vi "Operaciones Boleanas.vi"() -> ()   [LabVIEW 2022 SP3]
panel:
  out "AND COMPOUND":bool
  out "AND EN CASCADA":bool
  in  "Boton A 9":bool
  in  "Boton A 8":bool
  in  "Boton A 7":bool
  in  "Boton A 6":bool
  in  "Boton A 5":bool
  in  "Boton A 4":bool
  in  "Boton A 3":bool
  in  "Boton A 2":bool
  out "NAND":bool
  out "NOR":bool
  out "OR":bool
  out "AND":bool
  in  "Boton B":bool
  in  "Boton A":bool
  # "GATE AND Y OR"
  # "ESTA SOLUCION NOS DA UN RESULTADO PARA LO \n8 RESULTADOS , ES DECIR SI TODOS SON CERO LA \nCOMPUERTA AND TE DA CERO Y SI TODOS ESTAN \nEN 1 LA COMPUERTA AND TE DA 1"
  # "COMPOUND ARITMETIC"
  # "CON ESTA FUNCION PARA AHORRAR MEMORIA SE PUEDE USAR EL COMPUND \nARIMETMETIC QUE TE RESUMEN LAS OPERACIONES BOLEANAS QUE QUIERES\nEN UN SOLO BLOQUE"
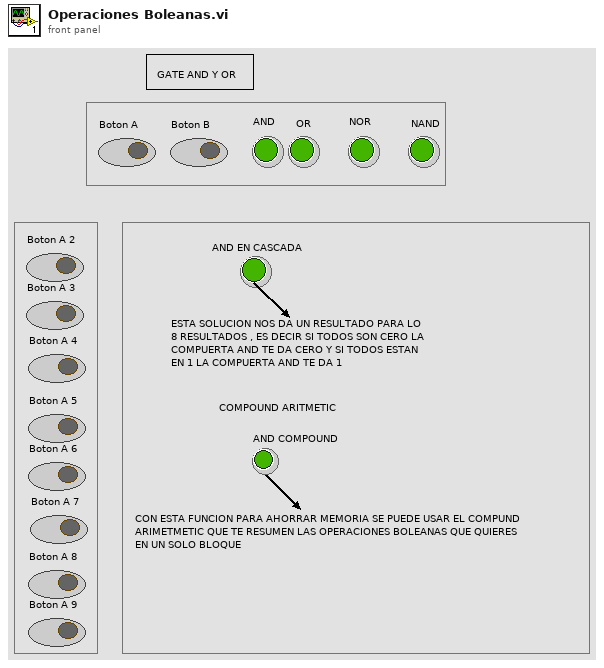
[diagram p1: front panel]
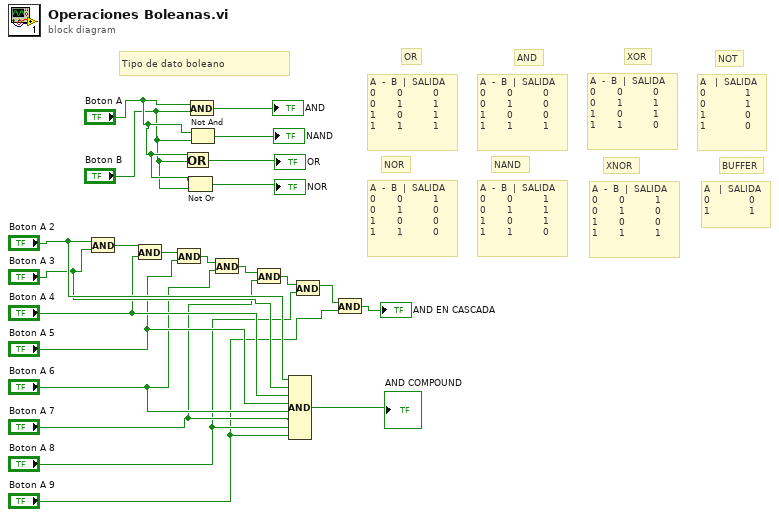
[diagram p0: block diagram]
diagram:
  # "A   |  SALIDA\n0             0\n1             1"
  # "BUFFER"
  # "A  -  B  |  SALIDA\n0       0          1\n0       1          0\n1       0          0\n1       1          1"
  # "XNOR"
  # "A  -  B  |  SALIDA\n0       0          1\n0       1          1\n1       0          1\n1       1          0"
  # "NAND"
  # "A  -  B  |  SALIDA\n0       0          1\n0       1          0\n1       0          0\n1       1          0"
  # "NOR"
  # "A   |  SALIDA\n0             1\n0             1\n1             0\n1             0"
  # "NOT"
  # "A  -  B  |  SALIDA\n0       0          0\n0       1          1\n1       0          1\n1       1          0"
  # "XOR"
  # "A  -  B  |  SALIDA\n0       0          0\n0       1          0\n1       0          0\n1       1          1"
  # "A  -  B  |  SALIDA\n0       0          0\n0       1          1\n1       0          1\n1       1          1"
  # "AND"
  # "OR"
  # "Tipo de dato boleano"
  n1 = And(x="Boton A 2", y="Boton A 3") -> (x .and. y?=w16:bool)
  n2 = And(x=w16, y="Boton A 4") -> (x .and. y?=w15:bool)
  n3 = And(x=w15, y="Boton A 5") -> (x .and. y?=w14:bool)
  n4 = Or(x="Boton A", y="Boton B") -> (x .or. y?=→"OR":bool)
  n5 = Not Or(1:"Boton B", 2:"Boton A") -> (0:→"NOR":bool)
  n6 = And(x="Boton A", y="Boton B") -> (x .and. y?=→"AND":bool)
  n7 = Not And(1:"Boton B", 2:"Boton A") -> (0:→"NAND":bool)
  n8 = And(x=w14, y="Boton A 6") -> (x .and. y?=w13:bool)
  n9 = And(x=w13, y="Boton A 7") -> (x .and. y?=w12:bool)
  n10 = Compound Arithmetic op=AND("Boton A 2", "Boton A 3", "Boton A 4", "Boton A 5", "Boton A 6", "Boton A 7", "Boton A 8", "Boton A 9") -> (→"AND COMPOUND":bool)
  n11 = And(x=w12, y="Boton A 8") -> (x .and. y?=w11:bool)
  n12 = And(x=w11, y="Boton A 9") -> (x .and. y?=→"AND EN CASCADA":bool)
